vi "i q sum.vi"(9 "input valid":bool=TRUE, 10 "data in":T1, 11 "data in":T1) -> (2 "output valid":bool, 3 "output cluster":T1)   [LabVIEW 2021]
doc: "sum 2 IQ datas (I+I =>I ; Q+Q =>Q ; overflow or overflow or +overflow => overflow"
uses:
  <instrlib>/_niInstr/DSP/v1/Shared/Public/IQ Data.ctl
  <vilib>/rvi/FXPMathLib/FxpAdd/XNode/nifxpmath_Add.xnode
  <vilib>/rvi/FXPMathLib/sim/FxpSim.dll
  <instrlib>/_niInstr/DSP/v1/Shared/niInstr DSP v1 Shared.lvlib
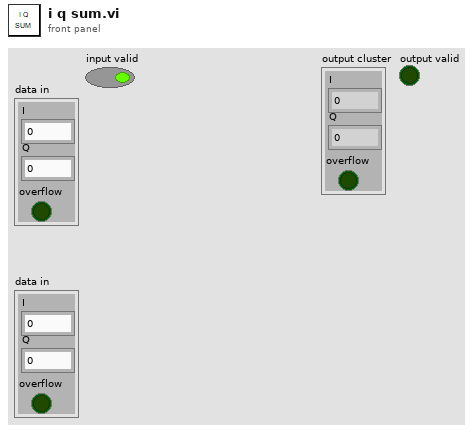
[diagram p1: front panel]
types:
  T1 = typedef "niInstr DSP v1 Shared.lvlib/IQ Data.ctl" = cluster{"I":fxp<+/-,18,1>, "Q":fxp<+/-,18,1>, "overflow":bool}
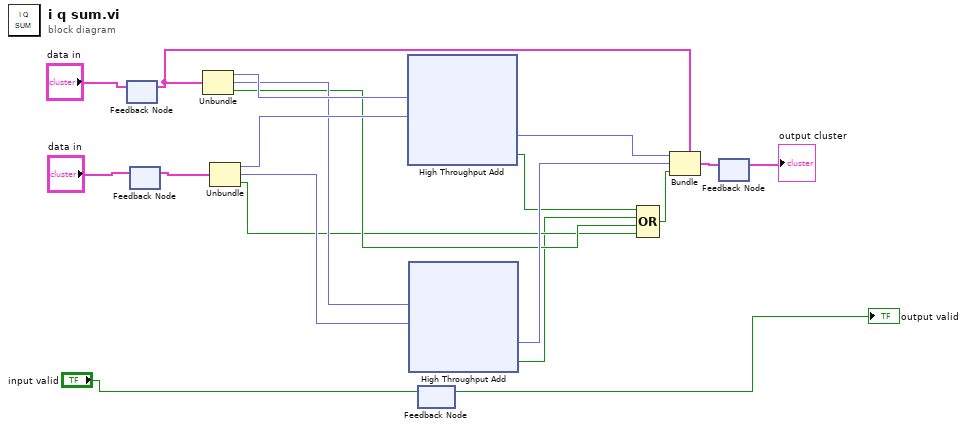
[diagram p0: block diagram]
diagram:
  n1 = feedback #1() -> (w1:T1)  [unwired: 1 in]
  n2 = feedback-in #1("data in") -> ()
  n3 = feedback-in #2("data in") -> ()
  n4 = feedback #2() -> (w7:T1)  [unwired: 1 in]
  n5 = Unbundle(w1) -> ("I"=w19:fxp<+/-,18,1>, "Q"=w17:fxp<+/-,18,1>, "overflow"=w13:bool)
  n6 = Unbundle(w7) -> ("I"=w18:fxp<+/-,18,1>, "Q"=w16:fxp<+/-,18,1>, "overflow"=w12:bool)
  n7 = xnode ("High Throughput Add")("x"=w19, "y"=w18) -> ("x+y"=w15:fxp<+/-,18,1>, "operation overflow"=w10:bool)
  n8 = xnode ("High Throughput Add")("x"=w17, "y"=w16) -> ("x+y"=w14:fxp<+/-,18,1>, "operation overflow"=w9:bool)
  n9 = feedback #3() -> (→"output valid":bool)  [unwired: 1 in]
  n10 = feedback-in #3("input valid") -> ()
  n11 = Compound Arithmetic op=OR(w10, w9, w13, w12) -> (w11:bool)
  n12 = Bundle(cluster=w1, "I"=w15, "Q"=w14, "overflow"=w11) -> (w3:T1)
  n13 = feedback #4() -> (→"output cluster":T1)  [unwired: 1 in]
  n14 = feedback-in #4(w3) -> ()
